vi "time to day.vi"(2 "time offset":timestamp, 3 "time in seconds":dbl) -> (0 "fractional day":dbl, 1 "nearest day":i32)   [LabVIEW 2019]
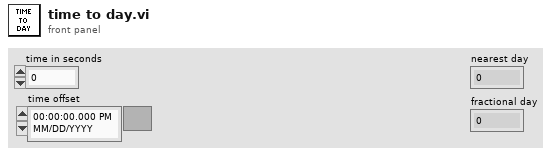
[diagram p1: front panel]
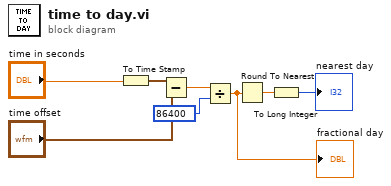
[diagram p0: block diagram]
diagram:
  n1 = To Time Stamp(1:"time in seconds") -> (0:w5:timestamp)
  n2 = Subtract(x=w5, y="time offset") -> (x-y=w6:dbl)
  n3 = Divide(x=w6, y=86400 ("Numeric")) -> (x/y=w7:dbl)
  "fractional day" <- w7
  n4 = Round To Nearest(number=w7) -> (nearest integer value=w8:dbl)
  n5 = To Long Integer(number=w8) -> (32bit integer=→"nearest day":i32)
